vi "PPL_TRAJ_Creation_Rel.vi"(6 "End Rotation Deg":dbl format="%#_13g", 11 "Max Velocity M/S":dbl=2.2 format="%17.3f") -> (0 "Path\nCreation\nError":bool, 1 "PathPlannerTrajectory":T16 {"States"."TargetHolonomicRotation"."SIN" format="%13.4f"; "States"."TargetHolonomicRotation"."COS" format="%13.4f"; "States"."TargetHolonomicRotation"."VALUE" format="%13.4f"; "States"."Heading"."SIN" format="%13.4f"; "States"."Heading"."COS" format="%13.4f"; "States"."Heading"."VALUE" format="%13.4f"; "States"."PositionMeters"."Y" format="%14.3f"; "States"."PositionMeters"."X" format="%14.3f"}, 2 "Trajectory State\nCount":i32, 3 "TotalTImeSecs":dbl)   [LabVIEW 2019]
uses:
  <vilib>/Rock Robotics/WPI/ThirdParty/MJansen/PathPlanner/PathPlanner24.lvlib
  <vilib>/Rock Robotics/WPI/ThirdParty/JAS_Junk/TrajLib/Trajectory_Library.lvlib
  <vilib>/Rock Robotics/WPI/ThirdParty/JAS_Junk/TrajLib/TypeDef/TRANSLATION2D.ctl
  <vilib>/Rock Robotics/WPI/ThirdParty/JAS_Junk/TrajLib/TypeDef/ROTATION2D.ctl
  <vilib>/Rock Robotics/WPI/ThirdParty/MJansen/PathPlanner/TypeDef/PathPlannerPathConstraints.ctl
  <vilib>/Rock Robotics/WPI/ThirdParty/MJansen/PathPlanner/TypeDef/PathPlannerTrajectoryState.ctl
  <vilib>/Rock Robotics/WPI/ThirdParty/MJansen/PathPlanner/TypeDef/PathPlannerTrajectory.ctl
  <vilib>/Rock Robotics/WPI/ThirdParty/JAS_Junk/TrajLib/TypeDef/POSE2D.ctl
  <vilib>/Rock Robotics/WPI/ThirdParty/MJansen/PathPlanner/TypeDef/PathPlannerRotationTarget.ctl
  <vilib>/Rock Robotics/WPI/ThirdParty/MJansen/PathPlanner/TypeDef/PathPlannerConstraintsZone.ctl
  <vilib>/Rock Robotics/WPI/ThirdParty/MJansen/PathPlanner/ENum/PathPlanner_CommandUtilType_ENUM.ctl
  <vilib>/Rock Robotics/WPI/ThirdParty/MJansen/PathPlanner/TypeDef/PathPlannerCommandUtil.ctl
  <vilib>/Rock Robotics/WPI/ThirdParty/MJansen/PathPlanner/TypeDef/PathPlannerEventMarker.ctl
  <vilib>/Rock Robotics/WPI/ThirdParty/MJansen/PathPlanner/TypeDef/PathPlannerGoalEndState.ctl
  <vilib>/Rock Robotics/WPI/ThirdParty/MJansen/PathPlanner/TypeDef/PathPlannerPathPoint.ctl
  <vilib>/Rock Robotics/WPI/ThirdParty/MJansen/PathPlanner/TypeDef/PathPlannerPath.ctl
  <vilib>/Rock Robotics/WPI/ThirdParty/MJansen/PathPlanner/TypeDef/PathPlannerWaypoint.ctl
  <vilib>/Rock Robotics/WPI/ThirdParty/MJansen/PathPlanner/TypeDef/PathPlannerPointTowardsZone.ctl
  <vilib>/Rock Robotics/WPI/ThirdParty/MJansen/PathPlanner/TypeDef/PathPlannerIdealStartingState.ctl
panel:
  in  "Current Pose SI 3":T1={"TRANSLATION"={"X"=3.0, "Y"=3.0}, "ROTATION"={"VALUE"=0.785, "COS"=0.707, "SIN"=0.707}} {"ROTATION"."SIN" format="%13.4f"; "ROTATION"."COS" format="%13.4f"; "ROTATION"."VALUE" format="%13.4f"; "TRANSLATION"."Y" format="%14.3f"; "TRANSLATION"."X" format="%14.3f"}
  in  "Current Pose SI 2":T1={"TRANSLATION"={"X"=2.0, "Y"=0.6}, "ROTATION"={"VALUE"=0.785, "COS"=0.707, "SIN"=0.707}} {"ROTATION"."SIN" format="%13.4f"; "ROTATION"."COS" format="%13.4f"; "ROTATION"."VALUE" format="%13.4f"; "TRANSLATION"."Y" format="%14.3f"; "TRANSLATION"."X" format="%14.3f"}
  out "PathPlannerPath":T4={"Reversed"=FALSE, "RotationTargets"=[], "ConstraintZones"=[], "EventMarkers"=[], "GlobalConstraints"={"MaxVelocityMps;"=0.0, "MaxAccelerationMpsSq;"=0.0, "MaxAngularVelRadPsEc;"=0.0, "MaxAngularAccRadPSecSq"=0.0, "Exists"=FALSE, "Unlimited"=FALSE, "NominalVoltageVolts"=1.0}, "GoalEndState"={"VelocityMPS"=0.0, "Rotation"={"VALUE"=0.0, "COS"=1.0, "SIN"=0.0}}, "AllPoints"=[], "Name"="", "Waypoints"=[], "PointTowardsZones"=[], "IdealStartingState"={"VelocityMPS"=0.0, "Rotation"={"VALUE"=0.0, "COS"=1.0, "SIN"=0.0}}, "IsChoreoPath"=FALSE, "PreventFlipping"=FALSE} {"IdealStartingState"."Rotation"."SIN" format="%13.4f"; "IdealStartingState"."Rotation"."COS" format="%13.4f"; "IdealStartingState"."Rotation"."VALUE" format="%13.4f"; "PointTowardsZones"."TargetPosition"."Y" format="%14.3f"; "PointTowardsZones"."TargetPosition"."X" format="%14.3f"; "PointTowardsZones"."RotationOffset"."SIN" format="%13.4f"; "PointTowardsZones"."RotationOffset"."COS" format="%13.4f"; "PointTowardsZones"."RotationOffset"."VALUE" format="%13.4f"; "Waypoints"."nextControl"."Y" format="%14.3f"; "Waypoints"."nextControl"."X" format="%14.3f"; "Waypoints"."anchor"."Y" format="%14.3f"; "Waypoints"."anchor"."X" format="%14.3f"; "Waypoints"."prevControl"."Y" format="%14.3f"; "Waypoints"."prevControl"."X" format="%14.3f"; "AllPoints"."RotationTarget"."rotation"."SIN" format="%13.4f"; "AllPoints"."RotationTarget"."rotation"."COS" format="%13.4f"; "AllPoints"."RotationTarget"."rotation"."VALUE" format="%13.4f"; "AllPoints"."Position"."Y" format="%14.3f"; "AllPoints"."Position"."X" format="%14.3f"; "GoalEndState"."Rotation"."SIN" format="%13.4f"; "GoalEndState"."Rotation"."COS" format="%13.4f"; "GoalEndState"."Rotation"."VALUE" format="%13.4f"; "RotationTargets"."rotation"."SIN" format="%13.4f"; "RotationTargets"."rotation"."COS" format="%13.4f"; "RotationTargets"."rotation"."VALUE" format="%13.4f"}
  in  "End Pose  SI":T1={"TRANSLATION"={"X"=5.75, "Y"=4.4}, "ROTATION"={"VALUE"=1.57, "COS"=0.0, "SIN"=1.0}} {"ROTATION"."SIN" format="%13.4f"; "ROTATION"."COS" format="%13.4f"; "ROTATION"."VALUE" format="%13.4f"; "TRANSLATION"."Y" format="%14.3f"; "TRANSLATION"."X" format="%14.3f"}
  in  "Current Pose SI":T1={"TRANSLATION"={"X"=0.0, "Y"=0.0}, "ROTATION"={"VALUE"=0.0, "COS"=1.0, "SIN"=0.0}} {"ROTATION"."SIN" format="%13.4f"; "ROTATION"."COS" format="%13.4f"; "ROTATION"."VALUE" format="%13.4f"; "TRANSLATION"."Y" format="%14.3f"; "TRANSLATION"."X" format="%14.3f"}
  in  "End Velocity M/S":dbl format="%#_13g"
  in  "Start Angual Vel Rad/S":dbl format="%#_13g"
  in  "Start Y Vel M/S":dbl format="%#_13g"
  in  "Start X Vel M/S":dbl format="%#_13g"
  in  "MaxAngularAccel Radians.Sec^2":dbl=1.0 format="%17.3f"
  out "Trajectory":cluster{dbl[], dbl[]}(graph)
  in  "MaxAcceleration M/S^2":dbl=1.8 format="%17.1f"
  in  "MaxAngularVel  Radians/Sec":dbl=1.0 format="%17.3f"
  # "Create PathPlanner Path/Trajectory Sample"
  # "This VI is designed to be called by BEGIN.VI, but can be executed directly to test trajectory parameters."
  # "CREATED TRAJECTORY INFORMATION"
  # "PATH CONFIGURATION"
  # "PATH DEFINITION"
  # "There can be as many points as needed."
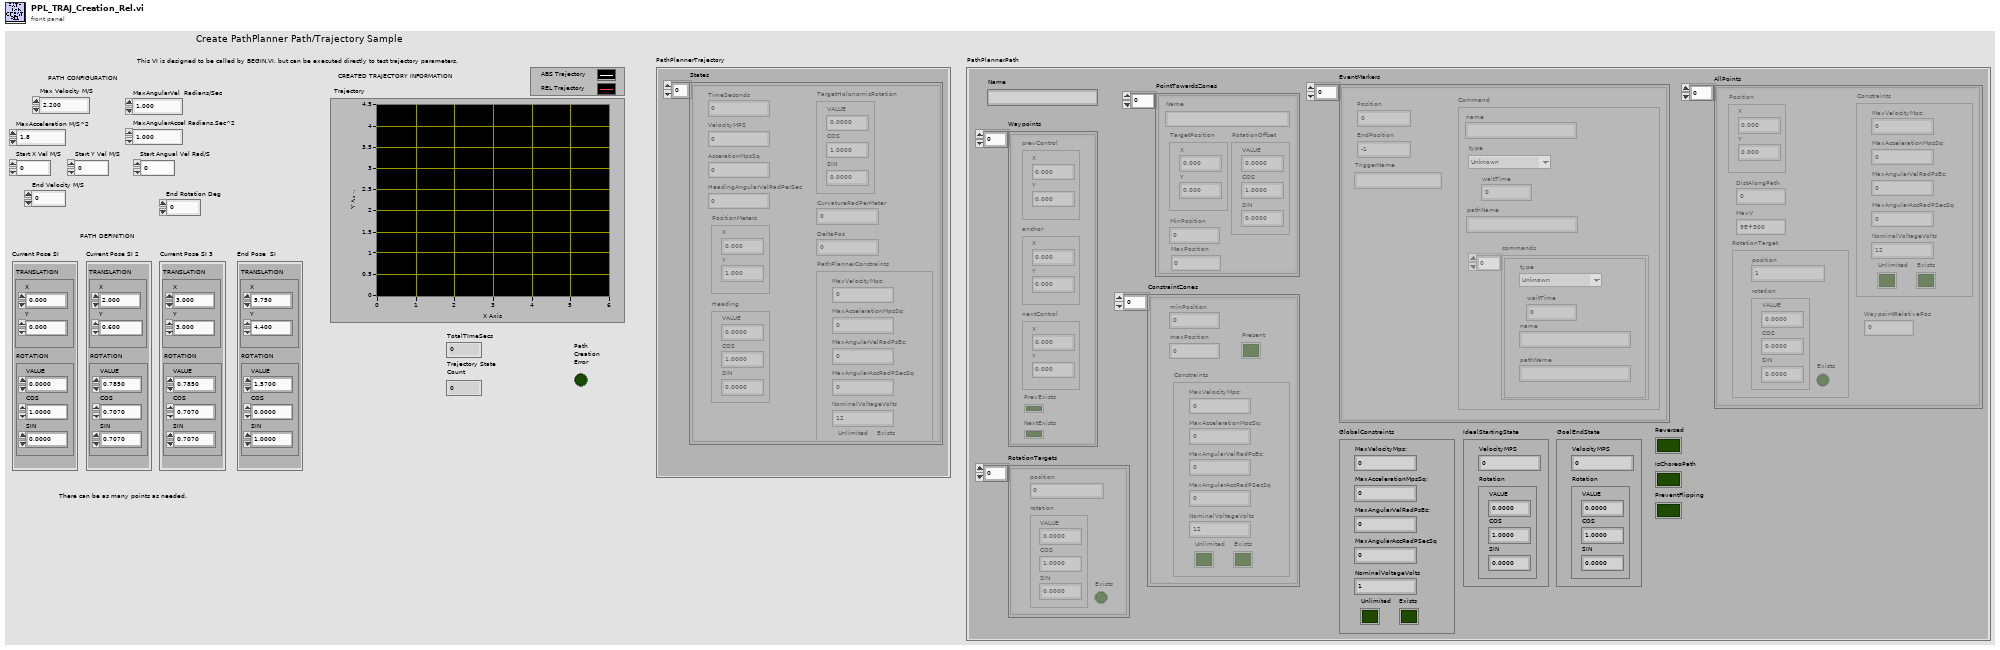
[diagram p1: front panel]
types:
  T1 = typedef "Trajectory_Library.lvlib/POSE2D.ctl" = cluster{"TRANSLATION":T2, "ROTATION":T3}
  T2 = typedef "Trajectory_Library.lvlib/TRANSLATION2D.ctl" = cluster{"X":dbl, "Y":dbl}
  T3 = typedef "Trajectory_Library.lvlib/ROTATION2D.ctl" = cluster{"VALUE":dbl, "COS":dbl, "SIN":dbl}
  T4 = typedef "PathPlanner24.lvlib/PathPlannerPath.ctl" = cluster{"Reversed":bool, "RotationTargets":T5[], "ConstraintZones":T6[], "EventMarkers":T8[], "GlobalConstraints":T7, "GoalEndState":T11, "AllPoints":T12[], "Name":string, "Waypoints":T13[], "PointTowardsZones":T14[], "IdealStartingState":T15, "IsChoreoPath":bool, "PreventFlipping":bool}
  T5 = typedef "PathPlanner24.lvlib/PathPlannerRotationTarget.ctl" = cluster{"position":dbl, "rotation":T3, "Exists":bool}
  T6 = typedef "PathPlanner24.lvlib/PathPlannerConstraintsZone.ctl" = cluster{"minPosition":dbl, "maxPosition":dbl, "Constraints":T7, "Present":bool}
  T7 = typedef "PathPlanner24.lvlib/PathPlannerPathConstraints.ctl" = cluster{"MaxVelocityMps;":dbl, "MaxAccelerationMpsSq;":dbl, "MaxAngularVelRadPsEc;":dbl, "MaxAngularAccRadPSecSq":dbl, "Exists":bool, "Unlimited":bool, "NominalVoltageVolts":dbl}
  T8 = typedef "PathPlanner24.lvlib/PathPlannerEventMarker.ctl" = cluster{"Position":dbl, "Command":T9, "TriggerName":string, "EndPosition":dbl}
  T9 = typedef "PathPlanner24.lvlib/PathPlannerCommandUtil.ctl" = cluster{"waitTime":dbl, "name":string, "pathName":string, "commands":cluster{"type":T10, "waitTime":dbl, "name":string, "pathName":string}[], "type":T10}
  T10 = typedef "PathPlanner24.lvlib/PathPlanner_CommandUtilType_ENUM.ctl" = enum16{"Unknown", "Wait", "Named", "Path", "Sequential", "Parallel", "Race", "Deadline"}
  T11 = typedef "PathPlanner24.lvlib/PathPlannerGoalEndState.ctl" = cluster{"VelocityMPS":dbl, "Rotation":T3}
  T12 = typedef "PathPlanner24.lvlib/PathPlannerPathPoint.ctl" = cluster{"Position":T2, "DistAlongPath":dbl, "MaxV":dbl, "Constraints":T7, "RotationTarget":T5, "WaypointRelativePos":dbl}
  T13 = typedef "PathPlanner24.lvlib/PathPlannerWaypoint.ctl" = cluster{"prevControl":T2, "anchor":T2, "nextControl":T2, "PrevExists":bool, "NextExists":bool}
  T14 = typedef "PathPlanner24.lvlib/PathPlannerPointTowardsZone.ctl" = cluster{"RotationOffset":T3, "Name":string, "TargetPosition":T2, "MinPosition":dbl, "MaxPosition":dbl}
  T15 = typedef "PathPlanner24.lvlib/PathPlannerIdealStartingState.ctl" = cluster{"VelocityMPS":dbl, "Rotation":T3}
  T16 = typedef "PathPlanner24.lvlib/PathPlannerTrajectory.ctl" = cluster{"States":T17[]}
  T17 = typedef "PathPlanner24.lvlib/PathPlannerTrajectoryState.ctl" = cluster{"TimeSeconds":dbl, "VelocityMPS":dbl, "AccerationMpsSq":dbl, "HeadingAngularVelRadPerSec":dbl, "PositionMeters":T2, "Heading":T3, "TargetHolonomicRotation":T3, "CurvatureRadPerMeter":dbl, "PathPlannerConstraints":T7, "DeltaPos":dbl}
  T18 = typedef "Trajectory_Library.lvlib/CHASSIS_SPEEDS.ctl" = cluster{"vX":dbl, "vY":dbl, "vOmega":dbl}
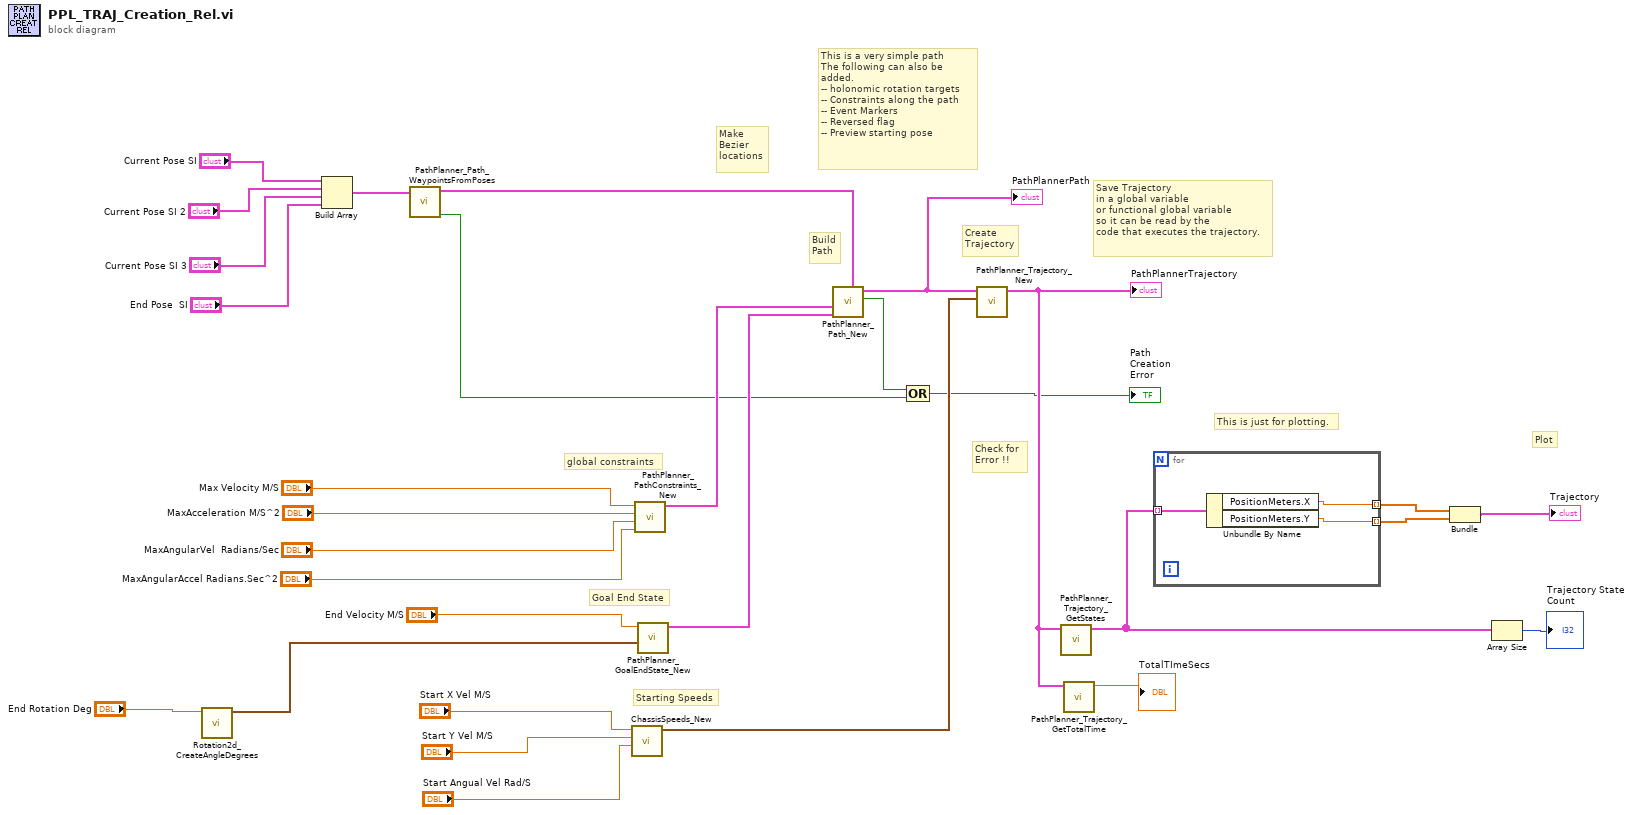
[diagram p0: block diagram]
diagram:
  # "This is just for plotting."
  # "This is a very simple path\nThe following can also be\nadded.\n-- holonomic rotation targets\n-- Constraints along the path\n-- Event Markers\n-- Reversed flag\n-- Preview starting pose"
  # "Plot"
  # "Save Trajectory\nin a global variable\nor functional global variable\nso it can be read by the \ncode that executes the trajectory."
  # "Create\nTrajectory"
  # "Check for\nError !!"
  # "Starting Speeds"
  # "Goal End State"
  # "global constraints"
  # "Make\nBezier\nlocations"
  # "Build\nPath"
  n1 = call <vilib>:"Rotation2d_CreateAngleDegrees.vi"("Angle_Degrees"="End Rotation Deg") -> ("ROTATION"=w2:T3)  [unwired: 10 in]
  n2 = Build Array("Current Pose SI", "Current Pose SI 2", "Current Pose SI 3", "End Pose  SI") -> (w6:T1[])
  n3 = call <vilib>:"PathPlanner_Path_WaypointsFromPoses.vi"("Poses"=w6) -> ("Error"=w4:bool, "Waypoints"=w5:T13[])  [unwired: 9 in]
  n4 = call <vilib>:"ChassisSpeeds_New.vi"("vAngular"="Start Angual Vel Rad/S", "vY"="Start Y Vel M/S", "vX"="Start X Vel M/S") -> ("CHASSIS"=w29:T18)  [unwired: 8 in]
  n5 = call <vilib>:"PathPlanner_PathConstraints_New.vi"("MaxAngularAccRadPSecSq"="MaxAngularAccel Radians.Sec^2", "MaxAngularVelRadPsEc;"="MaxAngularVel  Radians/Sec", "MaxAccelerationMpsSq;"="MaxAcceleration M/S^2", "MaxVelocityMps;"="Max Velocity M/S") -> ("PathPlannerConstraints"=w22:T7)  [unwired: 7 in]
  n6 = call <vilib>:"PathPlanner_GoalEndState_New.vi"("Rotation"=w2, "VelocityMPS"="End Velocity M/S") -> ("GoalEndState"=w24:T11)  [unwired: 9 in]
  n7 = call <vilib>:"PathPlanner_Path_New.vi"("Waypoints"=w5, "GoalEndState"=w24, "GlobalConstraints"=w22) -> ("Error"=w1:bool, "PathPlannerPath"=w25:T4)  [unwired: 7 in]
  "PathPlannerPath" <- w25
  n8 = Compound Arithmetic op=OR(w1, w4) -> (→"Path\nCreation\nError":bool)
  n9 = call <vilib>:"PathPlanner_Trajectory_New.vi"("StartingSpeeds"=w29, "Path"=w25) -> ("PathPlannerTrajectory"=w17:T16)  [unwired: 8 in, 1 out]
  "PathPlannerTrajectory" <- w17
  n10 = call <vilib>:"PathPlanner_Trajectory_GetStates.vi"("PathPlannerTrajectory"=w17) -> ("PathPlannerStates"=w18:T17[])  [unwired: 10 in]
  n11 = call <vilib>:"PathPlanner_Trajectory_GetTotalTime.vi"("PathPlannerTrajectory"=w17) -> ("TotalTimeSeconds"=→"TotalTImeSecs":dbl)  [unwired: 10 in]
  n12 = for {
    tunnel: [w33] -> w20 mode=indexing
    tunnel: [w32] -> w21 mode=indexing
    tunnel: w18 -> [w31] mode=indexing
    n13 = Unbundle By Name(w31) -> ("PositionMeters.X"=w33:dbl, "PositionMeters.Y"=w32:dbl)
  }
  n14 = Bundle(w20, w21) -> (→"Trajectory":cluster{dbl[], dbl[]})  [unwired: 1 in]
  n15 = Array Size(array=w18) -> (size(s)=→"Trajectory State\nCount":i32)
